vi "ParseLogError.vi"(8 "error in (no error)":errorcluster, 11 "message body":variant) -> (0 "error out":errorcluster, 3 "error string":string)   [LabVIEW 2017, in "TraceLogger.lvlib"]
uses:
  <vilib>/addons/TraceLogger/TraceLogger.lvlib
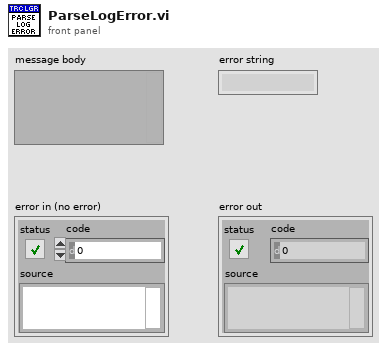
[diagram p1: front panel]
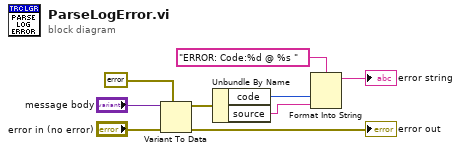
[diagram p0: block diagram]
diagram:
  n1 = Variant To Data(error in="error in (no error)", type=errorcluster {"status"=FALSE, "code"=0, "source"=""} ("error out"), Variant="message body") -> (data=w2:errorcluster, error out=→"error out":errorcluster)
  n2 = Unbundle By Name(w2) -> ("code"=w3:i32, "source"=w5:string)
  n3 = Format Into String(format string="ERROR: Code:%d @ %s ", w3, w5) -> (resulting string=→"error string":string)  [unwired: 2 in, 1 out]
